vi "dvp Vi Get Stream State.vi"(10 "pStreamState":u32(ring) items=["STATE_STOPED", "STATE_PAUSED", "STATE_STARTED"], 11 "handle":u32) -> (2 "pStreamState out":u32(ring) items=["STATE_STOPED", "STATE_PAUSED", "STATE_STARTED"], 3 "function return":u32(ring))   [LabVIEW 2018, in "LabViewDVPCamera.lvlib"]
doc: "LabviewDvp2Api dvpStatus dvpViGetStreamState(dvpHandle handle, dvpStreamState *pStreamState);"
uses:
  LabViewDVPCamera.lvlib
  LabViewDVPCamera/LabViewDVPCamera.dll
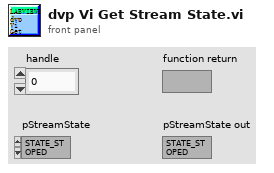
[diagram p1: front panel]
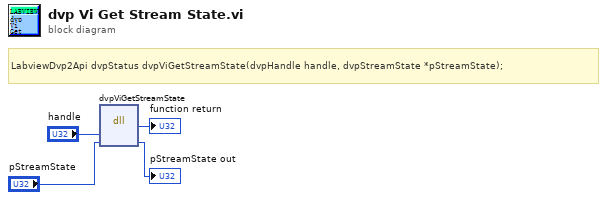
[diagram p0: block diagram]
diagram:
  # "LabviewDvp2Api dvpStatus dvpViGetStreamState(dvpHandle handle, dvpStreamState *pStreamState);"
  n1 = dll-call lib="C:/Program Files (x86)/DVP2 Labview cn 64/Sample/LabViewDVPCamera/LabViewDVPCamera.*" fn="dvpViGetStreamState"("handle"="handle", "pStreamState"="pStreamState") -> (→"function return":u32, "pStreamState"=→"pStreamState out":u32)  [unwired: 4 in, 2 out]
